vi "Refnums.vi"() -> ()   [LabVIEW 2015]
panel:
  in  "Indexer":string="Indexer"
  in  "ShooterWheel2":string="ShooterWheel2"
  in  "ShooterWheel1":string="ShooterWheel1"
  in  "Gunner":string="Gunner"
  in  "Drive":string="Drive"
  in  "PWM 0":string="Left1"
  in  "PWM 1":string="Left2"
  in  "PWM 2":string="Left3"
  in  "PWM 5":string="Right3"
  in  "PWM 3":string="Right1"
  in  "PWM 4":string="Right2"
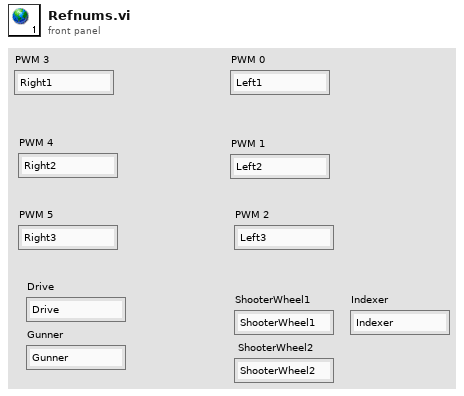
[diagram p1: front panel]
diagram:
